vi "Read Scalar Boolean.vi"(8 "error in (no error)":errorcluster, 11 "pointer in":u64) -> (0 "error out":errorcluster, 2 "value":bool, 3 "pointer out":u64)   [LabVIEW 2013, in "Linux RT IPC.lvlib" / "Shared Memory.lvlib"]
uses:
  Shared Memory.lvlib
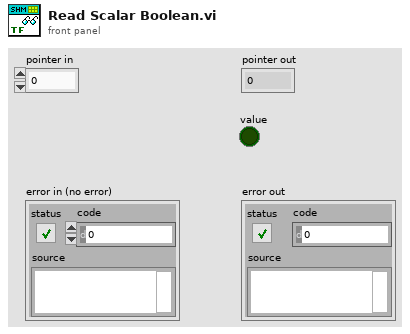
[diagram p1: front panel]
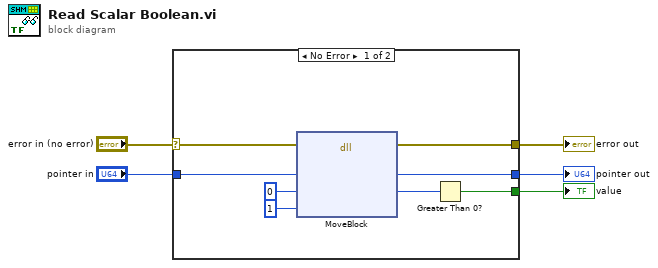
[diagram p0: block diagram]
diagram:
  n1 = case shown="No Error" "error in (no error)" {
    selector: "error in (no error)" -> [w10 w15]
    tunnel: [w8 w15] -> w5
    tunnel: "pointer in" -> [w9 w14]
    tunnel: [w6 w14] -> w2
    tunnel: [w13 _] -> w1
    frame No Error {
      n2 = dll-call lib="LabVIEW" fn="MoveBlock"(error in=w10, "pointer"=w9, "data"=u8 0, "size"=u64 1) -> (error out=w8:errorcluster, "pointer"=w6:u64, "data"=w7:u8)  [unwired: 4 in, 1 out]
      n3 = Greater Than 0?(x=w7) -> (x > 0?=w13:bool)
    }
    frame Error {
    }
  }
  "error out" <- w5
  "pointer out" <- w2
  "value" <- w1
